vi "1_SimpleDemo_MHHisto.vi"() -> ()   [LabVIEW 2010]
uses:
  _lib/PQ/MultiHarp/mhlib_x86_x64_UIThread.llb/MH_DllPath_global.vi
  _lib/PQ/MultiHarp/MH_RefSource.ctl
  _lib/PQ/MultiHarp/MH_LibVersion_global.vi
  _lib/PQ/MultiHarp/MH_MeasMode.ctl
panel:
  in  "EnableInputDeadTime":bool caption="Enable DeadTime"
  in  "InputDeadTime":i32=1000 caption="DeadTime [ps]" min=800 max=160000 step=1
  in  "Trg.Edge":i32(ring) items=["falling", "rising"]
  in  "Trg.Level":i32=-100 caption="Trg.Level [mV]" min=-1200 max=1200 step=1
  in  "Offset":i32 caption="Offset [ps]" min=-99999 max=99999 step=1
  in  "Enable":bool=TRUE
  in  "EnableSyncDeadTime":bool caption="Enable DeadTime"
  in  "SyncDeadTime":i32=1000 caption="SyncDeadTime [ps]" min=800 max=160000 step=1
  in  "SyncTrg.Edge":i32(ring) items=["falling", "rising"]
  in  "SyncTrg.Level":i32=-100 caption="SyncTrg.Level [mV]" min=-1200 max=1200 step=1
  in  "SyncOffset":i32 caption="SyncOffset [ps]" min=-99999 max=99999 step=1
  in  "SyncDivider":i32(ring)=1 items=["1"=1, "2"=2, "4"=4, "8"=8, "16"=16]
  in  "Binning":i32(ring) caption="Resolution [ps]" items=["80", "160", "320", "640", "1280", "2560", "5120", "10240", "20480", "40960", "81920", "163840", "327680", "655360", "1310720", "2621440", "5242880", "10485760", "20971520", "41943040", "83886080", "167772160", "335544320"]
  in  "HistoLength":i32(ring)=6 caption="Histo Length" items=["1024", "2048", "4096", "8192", "16384", "32768", "65536"]
  in  "Acqu.Time":i32=10000 caption="Acqu.Time [ms]" min=1 max=360000 step=1
  in  "GlobalOffset":i32 caption="GlobalOffset [ns]" min=0 max=100000000 step=1
  in  "OverflowLevel":u32=4294967295 min=1 step=1
  in  "StopOnOverflow":bool=TRUE
  out "HistoGraph":T1(graph)={0.0, "Resolution"=0.08, "Histogram"=array8x65536[524288 elements]}
  out "CountRates":i32[](array[numeric]) caption="Count Rates [cps]"
  out "SyncRate":i32 caption="Sync Rate [cps]"
  in  "stop":bool
  out "error out":errorcluster
  # "All Channels"
  # "Sync"
  # "Acquisition"
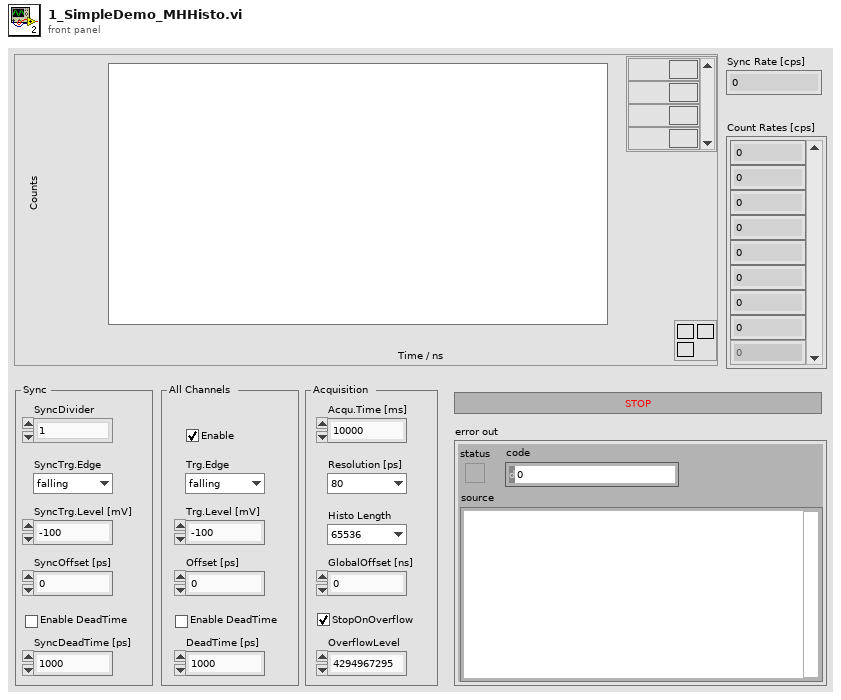
[diagram p1: front panel]
types:
  T1 = cluster{dbl, "Resolution":dbl, "Histogram":u32[][]}
  T2 = typedef "MH_MeasMode.ctl" = i32
  T3 = typedef "MH_RefSource.ctl" = enum16{"INTERNAL", "EXTERNAL_10MHZ", "WR_MASTER_GENERIC", "WR_SLAVE_GENERIC", "WR_GRANDM_GENERIC", "EXTN_GPS_PPS", "EXTN_GPS_PPS_UART", "WR_MASTER_MHARP", "WR_SLAVE_MHARP", "WR_GRANDM_MHARP"}
  T4 = typedef "MH_InitInfo.ctl" = cluster{"Library Version":string, "Serial No.":string, "Model":string, "Partnum":string, "Version":string, "features":i32, "nchannels":i32, "Base Resolution":dbl, "Bin Steps":i32}
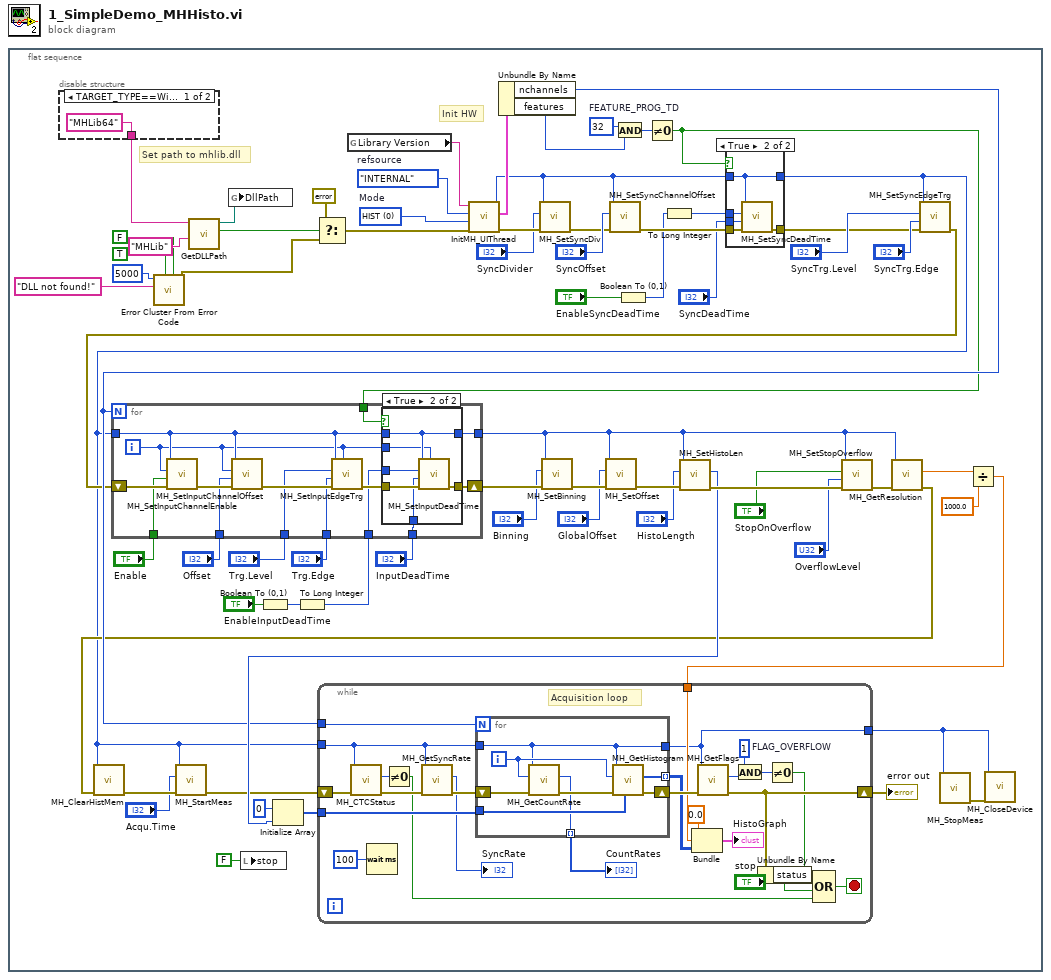
[diagram p0: block diagram]
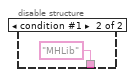
[diagram p3: hidden frame]
diagram:
  n1 = flat-sequence {
    frame #0 {
      w11 = 32  # FEATURE_PROG_TD
      w22 = T2 0 items=["HIST"=0, "T2"=2, "T3"=3]  # Mode
      w68 = MH_RefSource."INTERNAL"  # refsource
      # "Init HW"
      # "Set path to mhlib.dll"
      n2 = disable-structure shown="TARGET_TYPE==Windows, Default" {
        disable-tunnel: ["MHLib64" ("name or relative path") "MHLib" ("name or relative path")] -> w21
        frame condition #0 (active) {
        }
        frame condition #1 {
        }
      }
      n3 = call <vilib>:"Error Cluster From Error Code.vi"("is warning? (False)"=FALSE, "show call chain? (False)"=TRUE, "error message (\"\")"="DLL not found!" ("error message (\"\")"), "error code (0)"=5000) -> ("error out"=w67:errorcluster)  [unwired: 5 in]
      n4 = call "GetDLLPath.vi"("DllName_32bit"="MHLib" ("name or relative path"), "DllName_64bit"=w21) -> ("file exists?"=w65:bool, "DLLPath"=w64:path)  [unwired: 8 in]
      n5 = global write "MH_DllPath_global.vi" "DllPath"(w64) -> ()
      n6 = local write "stop"(FALSE ("stop")) -> ()
      n7 = Boolean To (0,1)(Boolean="EnableInputDeadTime") -> (0, 1=w7:i16)
      n8 = To Long Integer(number=w7) -> (32bit integer=w6:i32)
      n9 = Select(t=errorcluster {"status"=FALSE, "code"=0, "source"=""} ("error IO"), s=w65, f=w67) -> (s? t:f=w62:errorcluster)
      n10 = global read "MH_LibVersion_global.vi" "Library Version"() -> (w25:string)
      n11 = call "InitMH_UIThread.vi"("error in (no error)"=w62, "Mode"=w22, "refsource"=w68, "Library Version"=w25) -> ("error out"=w57:errorcluster, "Init Info"=w59:T4, "DevIdx"=w18:i32)  [unwired: 5 in]
      n12 = Unbundle By Name(w59) -> ("nchannels"=w39:i32, "features"=w13:i32)
      n13 = call "MH_SetSyncDiv.vi"("error in (no error)"=w57, "SyncDivider"="SyncDivider", "devidx"=w18) -> ("error out"=w56:errorcluster)  [unwired: 7 in, 1 out]
      n14 = call "MH_SetSyncChannelOffset.vi"("error in (no error)"=w56, "Offset"="SyncOffset", "devidx"=w18) -> ("error out"=w20:errorcluster)  [unwired: 7 in, 1 out]
      n15 = And(x=w11, y=w13) -> (x .and. y?=w12:i32)
      n16 = Boolean To (0,1)(Boolean="EnableSyncDeadTime") -> (0, 1=w16:i16)
      n17 = Not Equal To 0?(x=w12) -> (x != 0?=w5:bool)
      n18 = To Long Integer(number=w16) -> (32bit integer=w15:i32)
      n19 = case shown="True" w5 {
        tunnel: w20 -> [w69 w75]
        tunnel: [w69 w74] -> w19
        tunnel: w18 -> [w70 w71]
        tunnel: w15 -> [_ w73]
        tunnel: "SyncDeadTime" -> [_ w72]
        tunnel: [w70 w71] -> w10
        frame False {
        }
        frame True {
          n20 = call "MH_SetSyncDeadTime.vi"("error in (no error)"=w75, "deadtime"=w72, "on"=w73, "devidx"=w71) -> ("error out"=w74:errorcluster)  [unwired: 6 in, 1 out]
        }
      }
      n21 = call "MH_SetSyncEdgeTrg.vi"("error in (no error)"=w19, "edge"="SyncTrg.Edge", "level"="SyncTrg.Level", "devidx"=w10) -> ("error out"=w38:errorcluster)  [unwired: 6 in, 1 out]
      n22 = for {
        N: w39 -> [_]
        shift-right: [w116] -> w58
        shift-left: w38 -> [w125]
        tunnel: w10 -> [w117]
        tunnel: [w115] -> w33
        tunnel: "Enable" -> [w122]
        tunnel: "Offset" -> [w121]
        tunnel: "Trg.Edge" -> [w120]
        tunnel: "Trg.Level" -> [w119]
        tunnel: "InputDeadTime" -> [w113]
        tunnel: w6 -> [w112]
        tunnel: w5 -> [w111]
        i -> [w114]
        n23 = call "MH_SetInputChannelEnable.vi"("error in (no error)"=w125, "enable"=w122, "channel"=w114, "devidx"=w117) -> ("error out"=w124:errorcluster)  [unwired: 6 in, 1 out]
        n24 = call "MH_SetInputChannelOffset.vi"("error in (no error)"=w124, "Offset"=w121, "channel"=w114, "devidx"=w117) -> ("error out"=w123:errorcluster)  [unwired: 6 in, 1 out]
        n25 = call "MH_SetInputEdgeTrg.vi"("channel"=w114, "error in (no error)"=w123, "edge"=w120, "level"=w119, "devidx"=w117) -> ("error out"=w118:errorcluster)  [unwired: 5 in, 1 out]
        n26 = case shown="True" w111 {
          tunnel: w118 -> [w127 w133]
          tunnel: w117 -> [w126 w131]
          tunnel: [w127 w132] -> w116
          tunnel: [w126 w131] -> w115
          tunnel: w114 -> [_ w130]
          tunnel: w113 -> [_ w129]
          tunnel: w112 -> [_ w128]
          frame False {
          }
          frame True {
            n27 = call "MH_SetInputDeadTime.vi"("channel"=w130, "error in (no error)"=w133, "deadtime"=w129, "on"=w128, "devidx"=w131) -> ("error out"=w132:errorcluster)  [unwired: 5 in, 1 out]
          }
        }
      }
      n28 = call "MH_SetBinning.vi"("error in (no error)"=w58, "Binning"="Binning", "devidx"=w33) -> ("error out"=w54:errorcluster)  [unwired: 7 in, 1 out]
      n29 = call "MH_SetOffset.vi"("error in (no error)"=w54, "Offset"="GlobalOffset", "devidx"=w33) -> ("error out"=w52:errorcluster)  [unwired: 7 in, 1 out]
      n30 = call "MH_SetHistoLen.vi"("error in (no error)"=w52, "lencode"="HistoLength", "devidx"=w33) -> ("error out"=w51:errorcluster, "actuallen"=w44:i32)  [unwired: 6 in, 1 out]
      n31 = Initialize Array(u32 0, w44) -> (w43:u32[])
      n32 = call "MH_SetStopOverflow.vi"("error in (no error)"=w51, "stopcount"="OverflowLevel", "StopOnOverflow"="StopOnOverflow", "devidx"=w33) -> ("error out"=w34:errorcluster)  [unwired: 6 in, 1 out]
      n33 = call "MH_GetResolution.vi"("error in (no error)"=w34, "devidx"=w33) -> ("error out"=w31:errorcluster, "resolution"=w32:dbl)  [unwired: 7 in, 1 out]
      n34 = call "MH_ClearHistMem.vi"("error in (no error)"=w31, "devidx"=w10) -> ("error out"=w48:errorcluster)  [unwired: 8 in, 1 out]
      n35 = call "MH_StartMeas.vi"("error in (no error)"=w48, "tacq"="Acqu.Time", "devidx"=w10) -> ("error out"=w30:errorcluster)  [unwired: 7 in, 1 out]
      n36 = Divide(x=w32, y=1000.0) -> (x/y=w40:dbl)
      n37 = while {
        shift-right: [w90] -> w46
        shift-left: w30 -> [w101]
        tunnel: w10 -> [w97]
        tunnel: w39 -> [w100]
        tunnel: w43 -> [w92]
        tunnel: w40 -> [w84]
        tunnel: [w79] -> w24
        stop <- w91 stop-if-true
        w95 = 1  # FLAG_OVERFLOW
        # "Acquisition loop"
        n38 = call "MH_CTCStatus.vi"("error in (no error)"=w101, "devidx"=w97) -> ("error out"=w99:errorcluster, "ctcstatus"=w102:i32)  [unwired: 7 in, 1 out]
        n39 = Wait (ms)(milliseconds to wait=u32 100) -> ()  [unwired: 1 out]
        n40 = Not Equal To 0?(x=w102) -> (x != 0?=w81:bool)
        n41 = call "MH_GetSyncRate.vi"("error in (no error)"=w99, "devidx"=w97) -> ("error out"=w98:errorcluster, "syncrate"=→"SyncRate":i32)  [unwired: 7 in, 1 out]
        n42 = for {
          N: w100 -> [_]
          shift-right: [w110] -> w96
          shift-left: w98 -> [w109]
          tunnel: w97 -> [w106]
          tunnel: [w106] -> w79
          tunnel: w92 -> [w105]
          tunnel: [w104] -> w87 mode=indexing
          tunnel: [w103] -> w86 mode=indexing
          i -> [w107]
          n43 = call "MH_GetCountRate.vi"("error in (no error)"=w109, "Channel"=w107, "devidx"=w106) -> ("error out"=w108:errorcluster, "rate"=w104:i32)  [unwired: 6 in, 1 out]
          n44 = call "MH_GetHistogram.vi"("Chcount"=w105, "error in (no error)"=w108, "channel"=w107, "devidx"=w106) -> ("error out"=w110:errorcluster, "Histogram"=w103:u32[])  [unwired: 5 in, 1 out]
        }
        "CountRates" <- w87
        n45 = Bundle(0.0, w84, "Histogram"=w86) -> (→"HistoGraph":cluster{dbl, dbl, "Histogram":u32[][]})  [unwired: 1 in]
        n46 = call "MH_GetFlags.vi"("error in (no error)"=w96, "devidx"=w79) -> ("error out"=w90:errorcluster, "flags"=w93:i32)  [unwired: 7 in, 1 out]
        n47 = And(x=w95, y=w93) -> (x .and. y?=w94:i32)
        n48 = Unbundle By Name(w90) -> ("status"=w78:bool)
        n49 = Not Equal To 0?(x=w94) -> (x != 0?=w89:bool)
        n50 = Compound Arithmetic op=OR(w78, w89, "stop", w81) -> (w91:bool)
      }
      "error out" <- w46
      n51 = call "MH_StopMeas.vi"("devidx"=w24) -> ("error out"=w23:errorcluster)  [unwired: 9 in, 1 out]
      n52 = call "MH_CloseDevice.vi"("error in (no error)"=w23, "devidx"=w24) -> ()  [unwired: 8 in, 2 out]
    }
  }
